vi "34970_Module.vi"(5 "Agilent 34970A":bool=TRUE, 7 "Command":T2, 8 "error in (no error)":errorcluster, 10 "Canales":T1={"CH TEMPERATURAS"=["101", "102", "103", "104", "105", "106"], "CH PRESIONES"=["117", "118", "119", "120"], "CH CAUDALES"=["121"]}, 11 "VISA Agilent 34970A":refnum<visa-resource-name>="COM5") -> (0 "error out":errorcluster, 1 "CAUDALES":dbl[](array[numeric]), 2 "PRESIONES":dbl[](array[numeric]), 3 "TEMPERATURAS":dbl[](array[numeric]))   [LabVIEW 2017]
uses:
  34970_Module Control.ctl
  <instrlib>/Agilent 34970/Agilent 34970.lvlib
panel:
  out "Output Array":dbl[](array[numeric])=[0.0, 1.0, 1.0, 1.0, 0.0, 1.0, 0.0, 1.0, 1.0, 1.0, 1.0, 1.0, 1.0, 0.0, 1.0, 1.0, 0.0, 1.0, 1.0, 0.0]
  # "Output Data"
  # "Input Data"
  # "Los canales en rojo estan estropeados.\nLos canales de temperatur son PT100\ny se han de leer por parejas.\n\nNo queda por tanto ningún canal libre.\n\nEl caudal lo leeremos por el canal 21 o 22"
  # "S1_Temperatura(C)"
  # "S2_Temperatura(C)"
  # "S1_Presion(mbar)"
  # "S3_Temperatura(C)"
  # "S4_Temperatura(C)"
  # "S5_Temperatura(C)"
  # "S2_Presion(mbar)"
  # "S3_Presion(mbar)"
  # "S1_Temperatura(C)"
  # "S2_Temperatura(C)"
  # "S4_Presion(mbar)"
  # "S3_Temperatura(C)"
  # "S4_Temperatura(C)"
  # "S5_Temperatura(C)"
  # "Q1_Caudal(m3/h)"
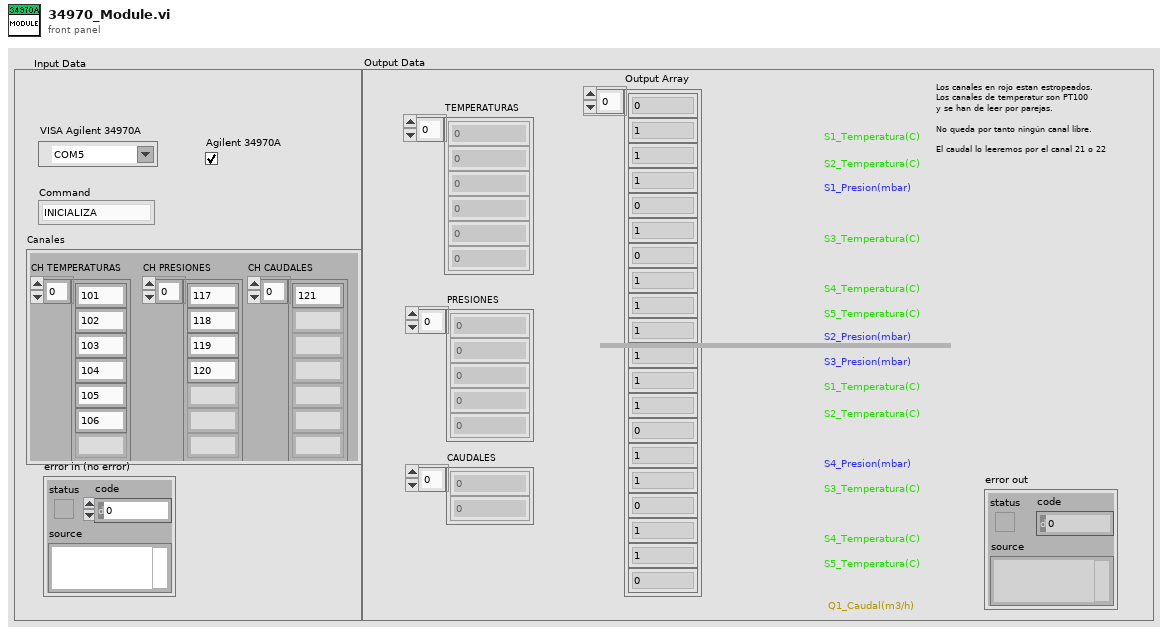
[diagram p1: front panel]
types:
  T1 = cluster{"CH TEMPERATURAS":string[], "CH PRESIONES":string[], "CH CAUDALES":string[]}
  T2 = typedef "34970_Module Control.ctl" = enum16{"INICIALIZA", "CONFIGURA CANALES", "LECTURA PT100", "LECTURA VOLTAJE", "LECTURA CORRIENTE", "SHUTDOWN"}
  T3 = cluster{"Timeout Value (10000)":u32, "Baud Rate (57600)":enum16{"1200", "2400", "4800", "9600", "19200", "38400", "57600", "115200"}, "Flow Control (1:XON/XOFF)":enum16{"None", "XON / XOFF", "RTS / CTS", "DTR / DSR"}}
  T4 = enum16{"Thermocouple", "Thermistor", "RTD", "4-Wire RTD", "Default (Last)"}
  T5 = enum16{"100 mV", "1 V", "10 V", "100 V", "300 V", "Auto", "Minimum", "Maximum"}
  T6 = enum16{"4 1/2", "5 1/2", "6 1/2", "Least", "Highest", "Default"}
  T7 = enum16{"10 mA", "100 mA", "1 A", "Auto", "Minimum", "Maximum"}
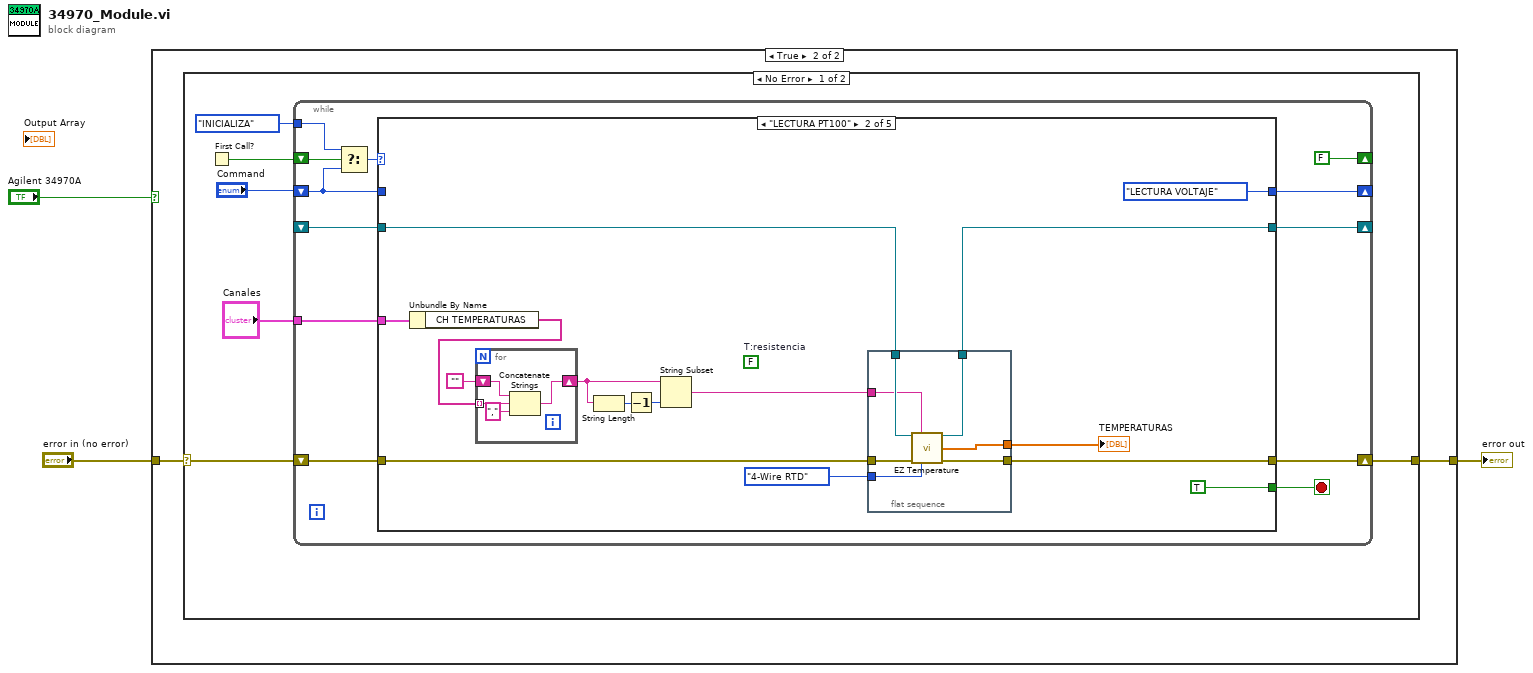
[diagram p0: block diagram]
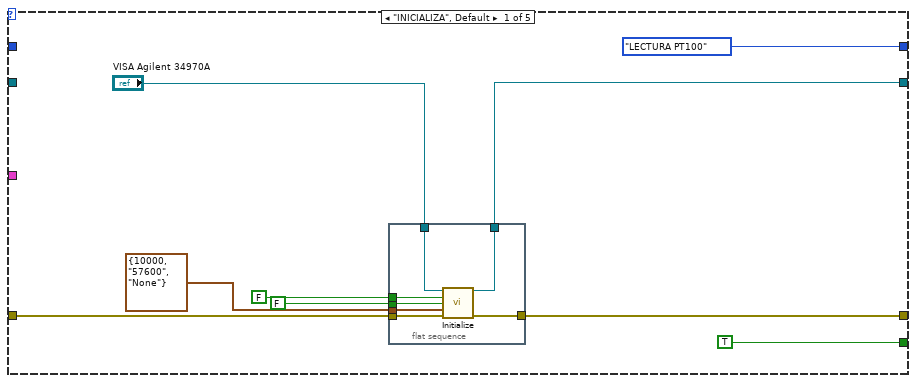
[diagram p3: hidden frame]
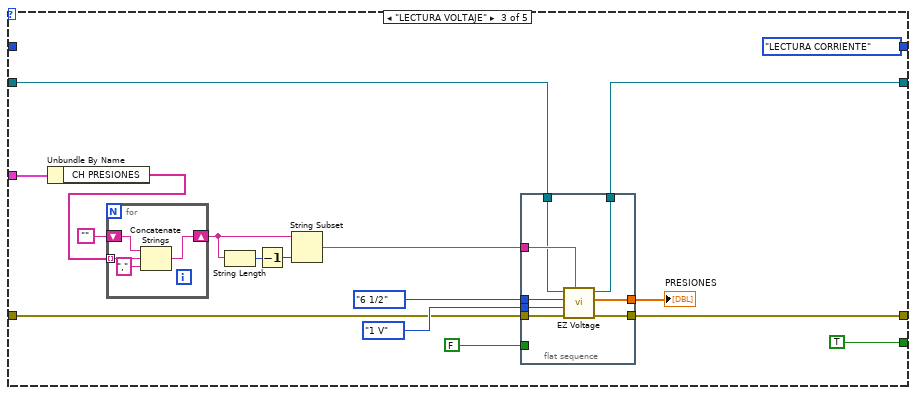
[diagram p4: hidden frame]
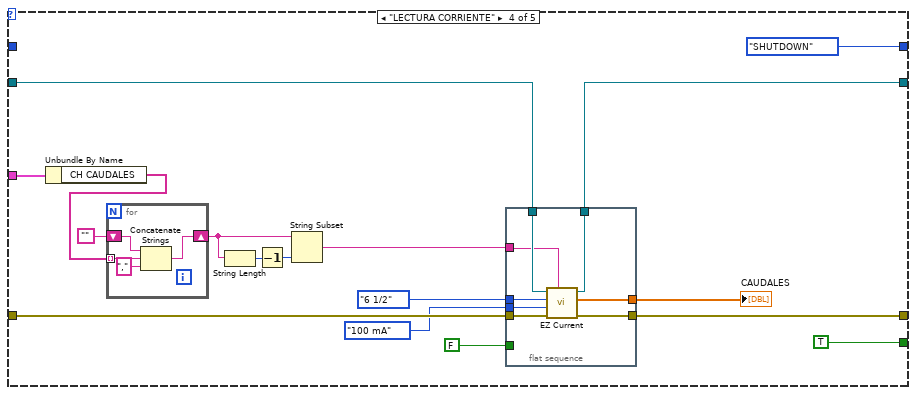
[diagram p5: hidden frame]
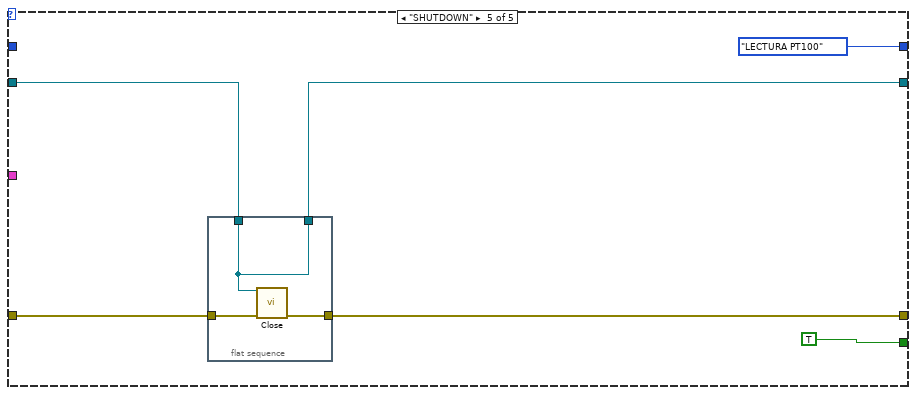
[diagram p6: hidden frame]
diagram:
  n1 = case shown="True" "Agilent 34970A" {
    tunnel: "error in (no error)" -> [w4 w6]
    tunnel: [w4 w5] -> w2
    frame False {
    }
    frame True {
      n2 = case shown="No Error" w6 {
        selector: w6 -> [w10 w134]
        tunnel: [w9 w134] -> w5
        frame No Error {
          n3 = First Call?() -> (First Call?: T/F=w12:bool)
          n4 = while {
            shift-right: [w18] -> _
            shift-left: "Command" -> [w19]
            shift-right: [w17] -> w9
            shift-left: w10 -> [w21]
            shift-right: [FALSE ("First Call?: T/F")] -> _
            shift-left: w12 -> [w24]
            tunnel: 34970_Module_Control."INICIALIZA" ("t") -> [w23]
            shift-right: [w15] -> _
            shift-left: _ -> [w16]
            tunnel: "Canales" -> [w13]
            stop <- w22 stop-if-true
            n5 = Select(t=w23, s=w24, f=w19) -> (s? t:f=w14:T2)
            n6 = case shown="\"LECTURA PT100\"" w14 {
              tunnel: [TRUE TRUE TRUE TRUE TRUE] -> w22
              tunnel: w21 -> [w30 w52 w71 w102 w130]
              tunnel: w19 -> [_ _ _ _ _]
              tunnel: [34970_Module_Control."LECTURA PT100" ("t") 34970_Module_Control."LECTURA VOLTAJE" ("t") 34970_Module_Control."LECTURA CORRIENTE" ("t") 34970_Module_Control."SHUTDOWN" ("t") 34970_Module_Control."LECTURA PT100" ("t")] -> w18
              tunnel: [w29 w46 w80 w109 w129] -> w17
              tunnel: w16 -> [_ w53 w70 w101 w126]
              tunnel: [w28 w45 w81 w110 w125] -> w15
              tunnel: w13 -> [_ w43 w68 w97 _]
              frame "INICIALIZA", Default {
                n7 = flat-sequence {
                  tunnel: "VISA Agilent 34970A" -> [w39]
                  tunnel: w30 -> [w38]
                  tunnel: [w37] -> w29
                  tunnel: [w40] -> w28
                  tunnel: T3 {"Timeout Value (10000)"=10000, "Baud Rate (57600)"=enum."57600", "Flow Control (1:XON/XOFF)"=enum."None"} ("Serial Port Configuration") -> [w36]
                  tunnel: FALSE ("Reset (T: Reset)") -> [w35]
                  tunnel: FALSE ("ID Query (T: Check)") -> [w34]
                  frame #0 {
                    n8 = call <instrlib>:"Initialize.vi"("VISA Resource Name"=w39, "ID Query (T: Check)"=w34, "Reset (T: Reset)"=w35, "Serial Port Configuration"=w36, "error in (no error)"=w38) -> ("VISA Resource Name Out"=w40:refnum<visa-resource-name>, "error out"=w37:errorcluster)  [unwired: 9 in]
                  }
                }
              }
              frame "LECTURA PT100" {
                (unwired) FALSE  # T:resistencia
                n9 = Unbundle By Name(w43) -> ("CH TEMPERATURAS"=w42:string[])
                n10 = for {
                  tunnel: w42 -> [w65] mode=indexing
                  shift-right: [w64] -> w51
                  shift-left: "" -> [w66]
                  n11 = Concatenate Strings(w66, w65, "," ("string")) -> (w64:string)
                }
                n12 = String Length(string=w51) -> (length=w49:i32)
                n13 = Decrement(x=w49) -> (x-1=w50:i32)
                n14 = String Subset(string=w51, length (rest)=w50) -> (substring=w47:string)  [unwired: 1 in]
                n15 = flat-sequence {
                  tunnel: w53 -> [w62]
                  tunnel: w52 -> [w58]
                  tunnel: w47 -> [w56]
                  tunnel: [w60] -> w46
                  tunnel: [w61] -> w45
                  tunnel: [w59] -> w44
                  tunnel: T4."4-Wire RTD" ("Transducer Type (4:Def-Last)") -> [w57]
                  frame #0 {
                    n16 = call <instrlib>:"EZ Temperature.vi"("VISA Resource Name"=w62, "Scan List (empty)"=w56, "error in (no error)"=w58, "Transducer Type (4:Def-Last)"=w57) -> ("VISA Resource Name Out"=w61:refnum<visa-resource-name>, "Output Array"=w59:dbl[], "error out"=w60:errorcluster)  [unwired: 9 in]
                  }
                }
                "TEMPERATURAS" <- w44
              }
              frame "LECTURA VOLTAJE" {
                n17 = Unbundle By Name(w68) -> ("CH PRESIONES"=w67:string[])
                n18 = for {
                  tunnel: w67 -> [w94] mode=indexing
                  shift-right: [w93] -> w79
                  shift-left: "" -> [w95]
                  n19 = Concatenate Strings(w95, w94, "," ("string")) -> (w93:string)
                }
                n20 = String Length(string=w79) -> (length=w77:i32)
                n21 = Decrement(x=w77) -> (x-1=w78:i32)
                n22 = String Subset(string=w79, length (rest)=w78) -> (substring=w72:string)  [unwired: 1 in]
                n23 = flat-sequence {
                  tunnel: [w84] -> w81
                  tunnel: [w88] -> w80
                  tunnel: FALSE ("AC/DC (F:DC)") -> [_]
                  tunnel: T6."6 1/2" ("Resolution (5:Default)") -> [w85]
                  tunnel: T5."1 V" ("Range (5:Auto)") -> [w86]
                  tunnel: w72 -> [w91]
                  tunnel: w71 -> [w87]
                  tunnel: w70 -> [w90]
                  tunnel: [w89] -> w69
                  frame #0 {
                    n24 = call <instrlib>:"EZ Voltage.vi"("Scan List (empty)"=w91, "error in (no error)"=w87, "Range (5:Auto)"=w86, "Resolution (5:Default)"=w85, "VISA Resource Name"=w90) -> ("error out"=w88:errorcluster, "Output Array"=w89:dbl[], "VISA Resource Name Out"=w84:refnum<visa-resource-name>)  [unwired: 4 in]
                  }
                }
                "PRESIONES" <- w69
              }
              frame "LECTURA CORRIENTE" {
                n25 = Unbundle By Name(w97) -> ("CH CAUDALES"=w96:string[])
                n26 = for {
                  tunnel: w96 -> [w123] mode=indexing
                  shift-right: [w122] -> w108
                  shift-left: "" -> [w124]
                  n27 = Concatenate Strings(w124, w123, "," ("string")) -> (w122:string)
                }
                n28 = String Length(string=w108) -> (length=w106:i32)
                n29 = Decrement(x=w106) -> (x-1=w107:i32)
                n30 = String Subset(string=w108, length (rest)=w107) -> (substring=w103:string)  [unwired: 1 in]
                n31 = flat-sequence {
                  tunnel: [w119] -> w110
                  tunnel: [w117] -> w109
                  tunnel: FALSE ("AC/DC (F:DC)") -> [_]
                  tunnel: w103 -> [w113]
                  tunnel: w102 -> [w118]
                  tunnel: w101 -> [w120]
                  tunnel: T6."6 1/2" ("Resolution (3:Least)") -> [w115]
                  tunnel: T7."100 mA" ("Range (3:Auto)") -> [w114]
                  tunnel: [w116] -> w98
                  frame #0 {
                    n32 = call <instrlib>:"EZ Current.vi"("Scan List (empty)"=w113, "error in (no error)"=w118, "Range (3:Auto)"=w114, "Resolution (3:Least)"=w115, "VISA Resource Name"=w120) -> ("error out"=w117:errorcluster, "Output Array"=w116:dbl[], "VISA Resource Name Out"=w119:refnum<visa-resource-name>)  [unwired: 4 in]
                  }
                }
                "CAUDALES" <- w98
              }
              frame "SHUTDOWN" {
                n33 = flat-sequence {
                  tunnel: w130 -> [w132]
                  tunnel: [w131] -> w129
                  tunnel: [w133] -> w125
                  tunnel: w126 -> [w133]
                  frame #0 {
                    n34 = call <instrlib>:"Close.vi"("VISA Resource Name"=w133, "error in (no error)"=w132) -> ("error out"=w131:errorcluster)  [unwired: 13 in]
                  }
                }
              }
            }
          }
        }
        frame Error {
        }
      }
    }
  }
  "error out" <- w2
